vi "CRYReport Pic Open Report Frame.vi"() -> (2 "pVIRef_Out":refnum<vi>)   [LabVIEW 2013]
uses:
  CRYWindow/DataView/VIEW/CRYView Global.vi
  CRYReport Global.vi
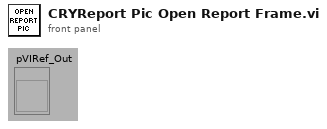
[diagram p1: front panel]
types:
  T1 = cluster{"sAction":string, "sType":string, "sQueueName":string, "sGraphName":string, "sData":string, "nData":i32, "pVIRef":refnum<vi>, "pSPRef":refnum<vi>}
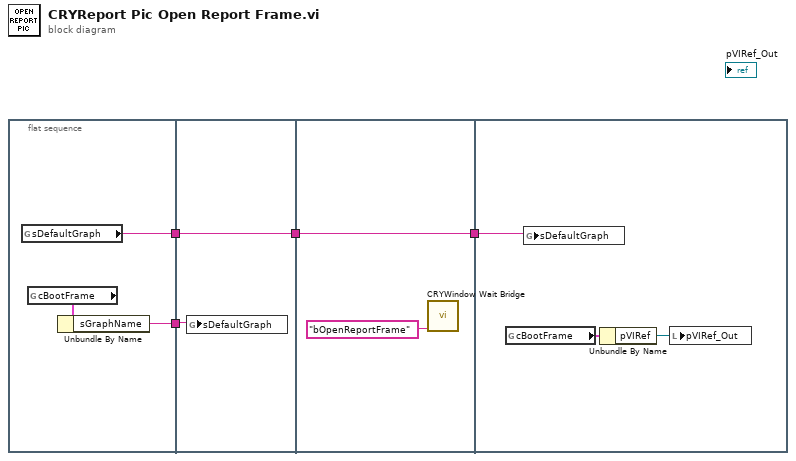
[diagram p0: block diagram]
diagram:
  n1 = flat-sequence {
    tunnel: [w6] -> w4
    tunnel: [w5] -> w1
    tunnel: w4 -> [w9]
    tunnel: [w8] -> w2
    tunnel: w1 -> [w8]
    tunnel: [w10] -> w3
    tunnel: w2 -> [w10]
    tunnel: w3 -> [w12]
    frame #0 {
      n2 = global read "CRYView Global.vi" "sDefaultGraph"() -> (w5:string)
      n3 = global read "CRYReport Global.vi" "cBootFrame"() -> (w7:T1)
      n4 = Unbundle By Name(w7) -> ("sGraphName"=w6:string)
    }
    frame #1 {
      n5 = global write "CRYView Global.vi" "sDefaultGraph"(w9) -> ()
    }
    frame #2 {
      n6 = call "CRYWindow Wait Bridge.vi"("sName"="bOpenReportFrame" ("Label Name")) -> ()  [unwired: 11 in]
    }
    frame #3 {
      n7 = global read "CRYReport Global.vi" "cBootFrame"() -> (w14:T1)
      n8 = global write "CRYView Global.vi" "sDefaultGraph"(w12) -> ()
      n9 = Unbundle By Name(w14) -> ("pVIRef"=w13:refnum<vi>)
      n10 = local write "pVIRef_Out"(w13) -> ()
    }
  }
